vi "Magazine_Execute.vi"() -> ()   [LabVIEW 2019]
uses:
  Globals/Magazine_Globals.vi
panel:
  in  "Unjam_Speed":dbl
  in  "Firing_Speed":dbl
  in  "Loading_Speed":dbl
  out "Magazine_Motor":dbl
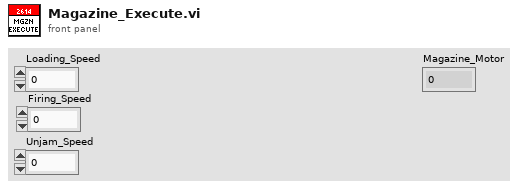
[diagram p1: front panel]
types:
  T1 = typedef "Magazine_Cluster.ctl" = cluster{"Control_States":enum16{"No-Op", "Loading", "Fire", "Unjam", "Manual"}, "Fire":bool, "Magazine_Throttle":dbl}
  T2 = enum16{"No-Op", "Loading", "Fire", "Unjam", "Manual"}
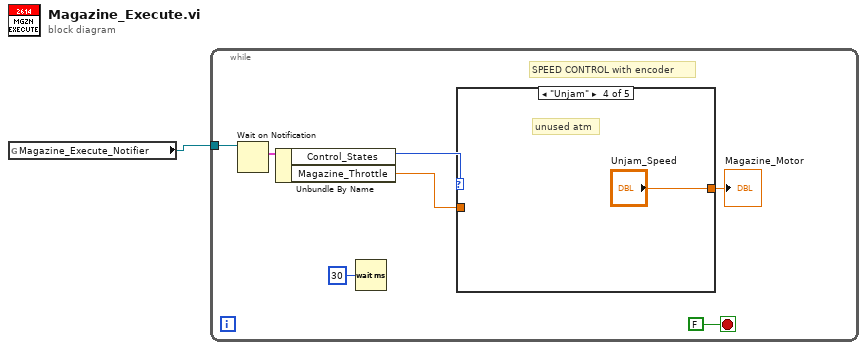
[diagram p0: block diagram]
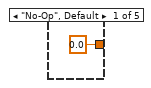
[diagram p2: hidden frame]
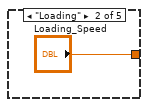
[diagram p3: hidden frame]
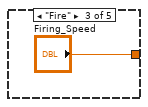
[diagram p4: hidden frame]
diagram:
  n1 = global read "Magazine_Globals.vi" "Magazine_Execute_Notifier"() -> (w1:refnum<notifier>)
  n2 = while {
    tunnel: w1 -> [w7]
    stop <- FALSE stop-if-true
    # "SPEED CONTROL with encoder"
    n3 = Wait on Notification(notifier=w7) -> (notification=w6:T1)  [unwired: 3 in, 3 out]
    n4 = Unbundle By Name(w6) -> ("Control_States"=w5:T2, "Magazine_Throttle"=w3:dbl)
    n5 = Wait (ms)(milliseconds to wait=u32 30) -> ()  [unwired: 1 out]
    n6 = case shown="\"Unjam\"" w5 {
      tunnel: w3 -> [_ _ _ _ w13]
      tunnel: [0.0 ("Magazine_Throttle") "Loading_Speed" "Firing_Speed" "Unjam_Speed" w13] -> w4
      frame "No-Op", Default {
      }
      frame "Loading" {
      }
      frame "Fire" {
      }
      frame "Unjam" {
        # "unused atm"
      }
      frame "Manual" {
      }
    }
    "Magazine_Motor" <- w4
  }
